vi "Redis@CreateSession__Parameter.vi"(1 "ParamterIn":string) -> (0 "ParamterOut":string)   [LabVIEW 2020]
panel:
  in  "RedisKey":string(combo)
  in  "Password":string(combo)
  in  "UserName":string(combo)
  in  "Port":string(combo)
  in  "Host":string(combo)
  in  "RedisSession":string(combo)
  in  "Confirm":bool
  # "RedisSession,Host:Port(,User:Password)\nRedisSession,RedisKey@Host:Port(,User:Password)"
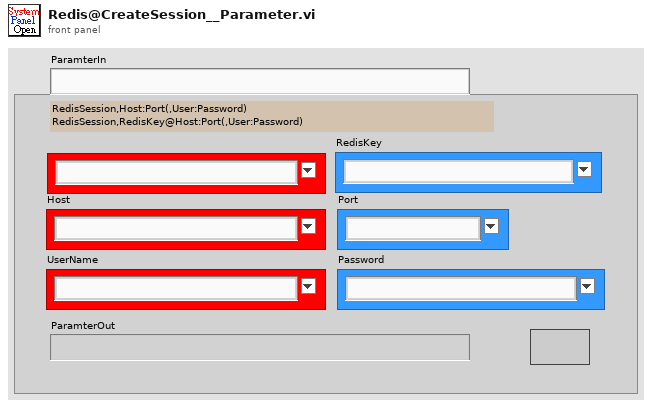
[diagram p1: front panel]
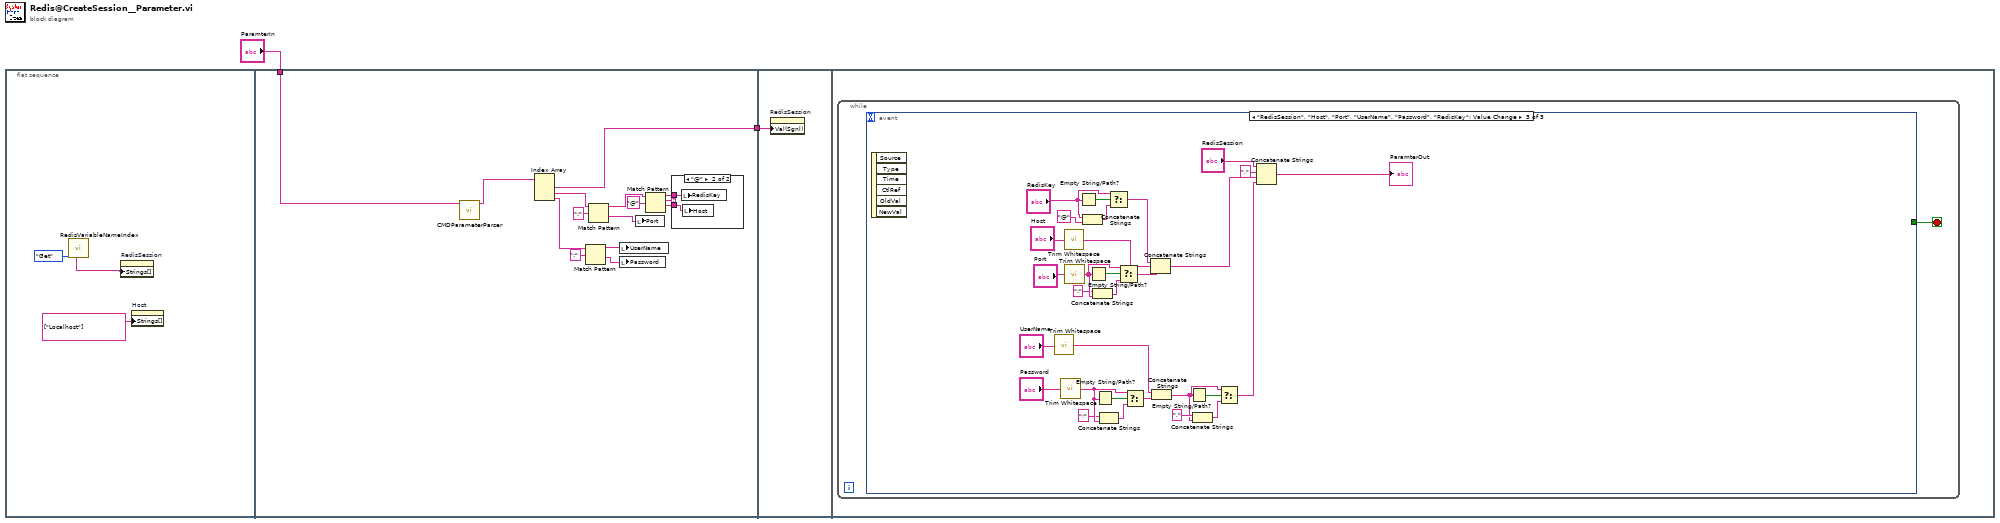
[diagram p0: block diagram]
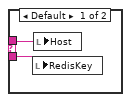
[diagram p2: hidden frame]
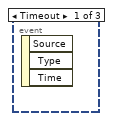
[diagram p3: hidden frame]
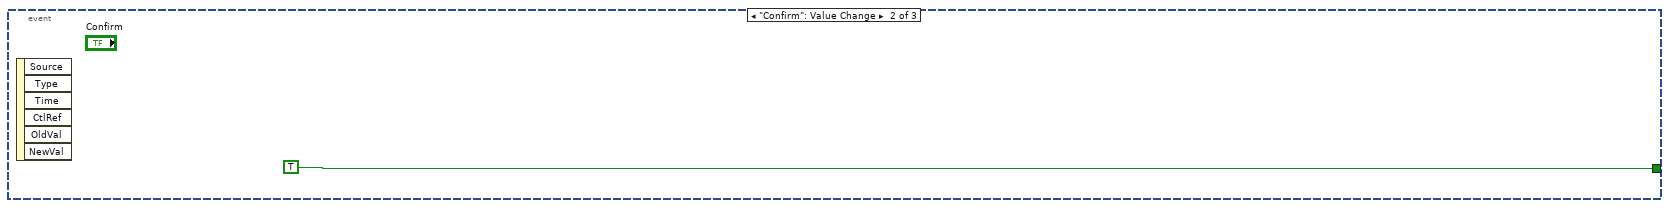
[diagram p4: hidden frame]
diagram:
  n1 = flat-sequence {
    tunnel: "ParamterIn" -> [w20]
    tunnel: [w18] -> w1
    tunnel: w1 -> [w25]
    frame #0 {
      n2 = call "RedisVariableNameIndex.vi"("OP"=enum16{"Add", "Init", "Get"}."Get") -> ("RedisSessionS"=w4:string[])  [unwired: 6 in, 4 out]
      n3 = property on="RedisSession" class="CmbBox"("Strings[]"=w4) -> ()  [unwired: 2 in, 2 out]
      n4 = property on="Host" class="CmbBox"("Strings[]"=string[] ["Localhost"] ("Strings []")) -> ()  [unwired: 2 in, 2 out]
    }
    frame #1 {
      n5 = call "CMDParameterParser.vi"("CMDParameter"=w20) -> ("Input"=w19:string[])  [unwired: 8 in, 2 out]
      n6 = Index Array(array=w19) -> (element #1=w18:string, element #2=w17:string, element #3=w11:string)  [unwired: 3 in]
      n7 = Match Pattern(string=w11, regular expression=":") -> (before substring=w10:string, after substring=w9:string)  [unwired: 1 in, 2 out]
      n8 = Match Pattern(string=w17, regular expression=":") -> (before substring=w14:string, after substring=w13:string)  [unwired: 1 in, 2 out]
      n9 = local write "UserName"(w10) -> ()
      n10 = local write "Password"(w9) -> ()
      n11 = local write "Port"(w13) -> ()
      n12 = Match Pattern(string=w14, regular expression="@") -> (before substring=w7:string, match substring=w8:string, after substring=w6:string)  [unwired: 1 in, 1 out]
      n13 = case shown="\"@\"" w8 {
        tunnel: w7 -> [w22 w24]
        tunnel: w6 -> [w21 w23]
        frame Default {
          n14 = local write "RedisKey"(w21) -> ()
          n15 = local write "Host"(w22) -> ()
        }
        frame "@" {
          n16 = local write "RedisKey"(w24) -> ()
          n17 = local write "Host"(w23) -> ()
        }
      }
    }
    frame #2 {
      n18 = property on="RedisSession" class="CmbBox"("Val(Sgnl)"=w25) -> ()  [unwired: 2 in, 2 out]
    }
    frame #3 {
      n19 = while {
        stop <- w26 stop-if-true
        n20 = event shown="[2] \"RedisSession\", \"Host\", \"Port\", \"UserName\", \"Password\", \"RedisKey\": Value Change" {
          selector: _ -> [_ _ _]
          dyn-events: _ -> [_ _ _]
          timeout: _ -> [_ _ _]
          tunnel: [_ TRUE _] -> w26
          event Timeout {
            n21 = event-data() -> ()  [unwired: 1 in, 3 out]
          }
          event "Confirm": Value Change {
            n22 = event-data() -> ()  [unwired: 1 in, 6 out]
          }
          event "RedisSession", "Host", "Port", "UserName", "Password", "RedisKey": Value Change {
            n23 = event-data() -> ()  [unwired: 1 in, 6 out]
            n24 = call <vilib>:"Trim Whitespace.vi"("string"="UserName") -> ("trimmed string"=w39:string)  [unwired: 1 in]
            n25 = call <vilib>:"Trim Whitespace.vi"("string"="Password") -> ("trimmed string"=w44:string)  [unwired: 1 in]
            n26 = call <vilib>:"Trim Whitespace.vi"("string"="Host") -> ("trimmed string"=w41:string)  [unwired: 1 in]
            n27 = call <vilib>:"Trim Whitespace.vi"("string"="Port") -> ("trimmed string"=w48:string)  [unwired: 1 in]
            n28 = Empty String/Path?(string/path="RedisKey") -> (empty?=w31:bool)
            n29 = Concatenate Strings("RedisKey", "@" ("string")) -> (w32:string)
            n30 = Empty String/Path?(string/path=w48) -> (empty?=w50:bool)
            n31 = Concatenate Strings(":" ("string"), w48) -> (w49:string)
            n32 = Empty String/Path?(string/path=w44) -> (empty?=w45:bool)
            n33 = Concatenate Strings(":" ("string"), w44) -> (w46:string)
            n34 = Select(t="RedisKey", s=w31, f=w32) -> (s? t:f=w30:string)
            n35 = Select(t=w48, s=w50, f=w49) -> (s? t:f=w42:string)
            n36 = Select(t=w44, s=w45, f=w46) -> (s? t:f=w40:string)
            n37 = Concatenate Strings(w30, w41, w42) -> (w38:string)
            n38 = Concatenate Strings(w39, w40) -> (w35:string)
            n39 = Empty String/Path?(string/path=w35) -> (empty?=w37:bool)
            n40 = Concatenate Strings("," ("string"), w35) -> (w34:string)
            n41 = Select(t=w35, s=w37, f=w34) -> (s? t:f=w33:string)
            n42 = Concatenate Strings("RedisSession", "," ("string"), w38, w33) -> (→"ParamterOut":string)
          }
        }
      }
    }
  }
